vi "WaveID.vi"() -> ()   [LabVIEW 2024]
panel:
  in  "with damping":waveform(dbl)(graph)={"t0"=timestamp(0 s since 1904-01-01), "dt"=2.2727272727272726e-05, "Y"=array[44000 elements]}
  in  "Simple wave":waveform(dbl)(graph)={"t0"=timestamp(0 s since 1904-01-01), "dt"=2.2727272727272726e-05, "Y"=array[44000 elements]}
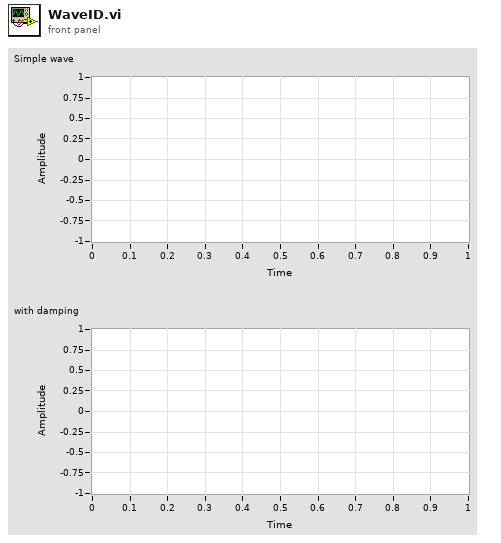
[diagram p1: front panel]
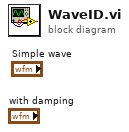
[diagram p0: block diagram]
diagram:
